vi "Radius_of_fi.vi"(1 "fi":dbl, 2 "e":dbl, 3 "a":dbl) -> (0 "r":dbl)   [LabVIEW 2020]
doc: "Calculate radius using r=a*(1-e^2)/(1+e*cos(fi) formula."
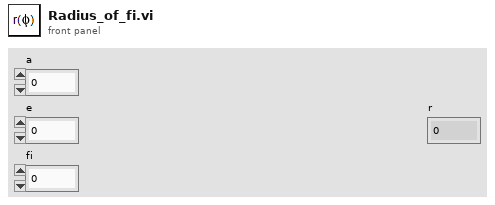
[diagram p1: front panel]
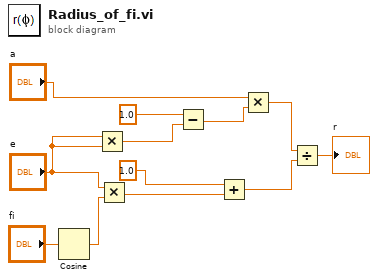
[diagram p0: block diagram]
diagram:
  n1 = Cosine(x="fi") -> (cos(x)=w7:dbl)
  n2 = Multiply(x="e", y="e") -> (x*y=w11:dbl)
  n3 = Multiply(x="e", y=w7) -> (x*y=w4:dbl)
  n4 = Subtract(x=1.0, y=w11) -> (x-y=w9:dbl)
  n5 = Add(x=1.0, y=w4) -> (x+y=w2:dbl)
  n6 = Multiply(x="a", y=w9) -> (x*y=w3:dbl)
  n7 = Divide(x=w3, y=w2) -> (x/y=→"r":dbl)
